vi "LoadStation.vi"(11 "Prog Data In":T1={"Station"=[], "Sensor List"=[], "Sensor Id"=[], "Parameters"=["PM10", "PM2.5", "ozon", "dwutlenek azotu", "dwutlenek siarki", "benzen", "tlenek węgla"], "Values"=[110, 75, 180, 200, 350, 21, 15]}) -> (0 "Error Out":errorcluster, 3 "Prog Data Out":T1={"Station"=[], "Sensor List"=[], "Sensor Id"=[], "Parameters"=["PM10", "PM2.5", "ozon", "dwutlenek azotu", "dwutlenek siarki", "benzen", "tlenek węgla"], "Values"=[110, 75, 180, 200, 350, 21, 15]})   [LabVIEW 2020]
doc: "This VI provide info about selected station by load file with last data or if file doesn't exist runs list of all stations to chose."
uses:
  Ctrls/ProgData.ctl
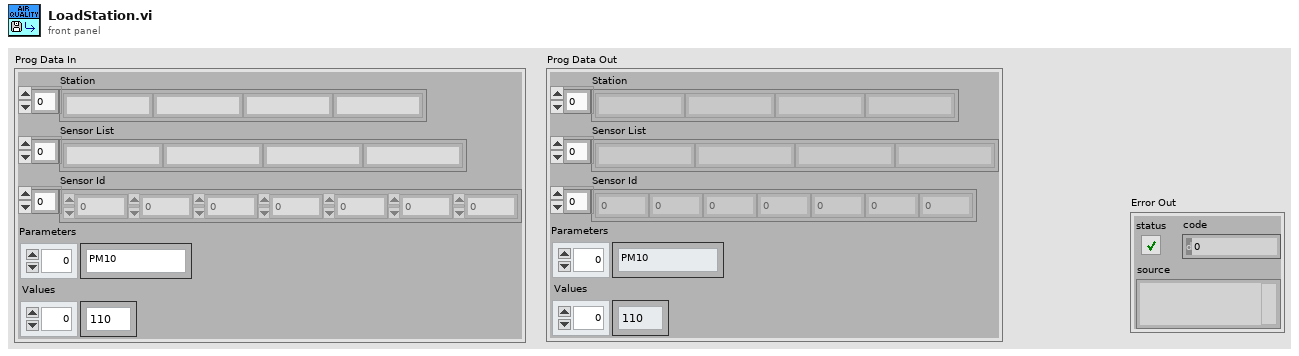
[diagram p1: front panel]
types:
  T1 = typedef "ProgData.ctl" = cluster{"Station":string[], "Sensor List":string[], "Sensor Id":dbl[], "Parameters":string[], "Values":i32[]}
  T2 = enum16{"open", "replace", "create", "open or create", "replace or create", "replace or create with confirmation"}
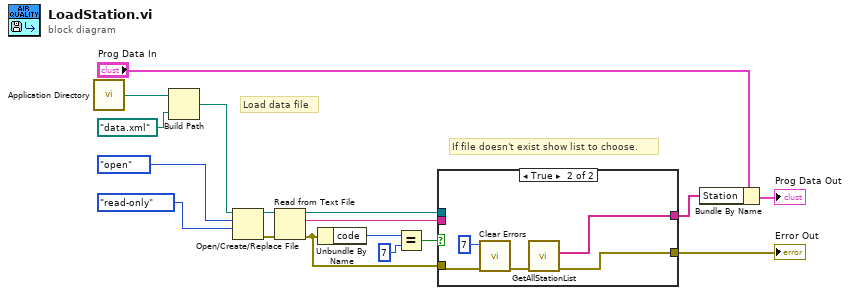
[diagram p0: block diagram]
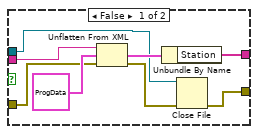
[diagram p2: hidden frame]
diagram:
  # "If file doesn't exist show list to choose."
  # "Load data file"
  n1 = call <vilib>:"Application Directory.vi"() -> ("Application Directory"=w11:path)
  n2 = Build Path(base path=w11, name or relative path=path "data.xml") -> (appended path=w10:path)
  n3 = Open/Create/Replace File(file path (use dialog)=w10, operation (0:open)=T2."open", access (0:read/write)=enum16{"read/write", "read-only", "write-only"}."read-only") -> (refnum out=w15:refnum<file>, error out=w14:errorcluster)  [unwired: 3 in, 1 out]
  n4 = Read from Text File(file (use dialog)=w15, error in=w14) -> (refnum out=w1:refnum<file>, text=w13:string, error out=w6:errorcluster)  [unwired: 2 in, 1 out]
  n5 = Unbundle By Name(w6) -> ("code"=w9:i32)
  n6 = Equal?(x=w9, y=7) -> (x = y?=w7:bool)
  n7 = case shown="True" w7 {
    tunnel: w13 -> [w25 _]
    tunnel: w6 -> [w23 w30]
    tunnel: [w19 w27] -> w5
    tunnel: [w21 w26] -> w2
    tunnel: w1 -> [w18 _]
    frame False {
      n8 = Unflatten From XML(xml string=w25, type=T1 {"Station"=[], "Sensor List"=[], "Sensor Id"=[], "Parameters"=["PM10", "PM2.5", "ozon", "dwutlenek azotu", "dwutlenek siarki", "benzen", "tlenek węgla"], "Values"=[110, 75, 180, 200, 350, 21, 15]}, error in (no error)=w23) -> (value=w22:T1, error out=w20:errorcluster)
      n9 = Unbundle By Name(w22) -> ("Station"=w21:string[])
      n10 = Close File(refnum=w18, error in=w20) -> (error out=w19:errorcluster)  [unwired: 1 out]
    }
    frame True {
      n11 = call <vilib>:"Clear Errors.vi"("error in (no error)"=w30, "specific error code to clear (0: all)"=7) -> ("error out"=w28:errorcluster)  [unwired: 4 in, 1 out]
      n12 = call "GetAllStationList.vi"("Error In"=w28) -> ("Error Out"=w27:errorcluster, "Station"=w26:string[])  [unwired: 9 in]
    }
  }
  "Error Out" <- w5
  n13 = Bundle By Name(cluster="Prog Data In", "Station"=w2) -> (→"Prog Data Out":T1)
